vi "OP500ZP_SEALING.vi"(8 "ERRIN":errorcluster caption="entrée d'erreur (pas d'erreur)") -> (0 "ERROUT":errorcluster caption="sortie d'erreur", 2 "SEALING_VALUE":dbl, 3 "IsOK?":bool)   [LabVIEW 2020]
uses:
  VG/VG_ATEQ.vi
  <instrlib>/HIOKI BT356X Series/HIOKI BT356X Series.lvlib
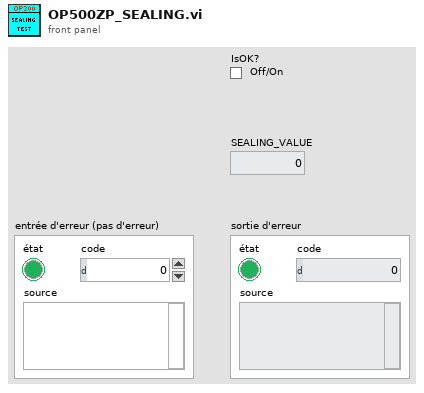
[diagram p1: front panel]
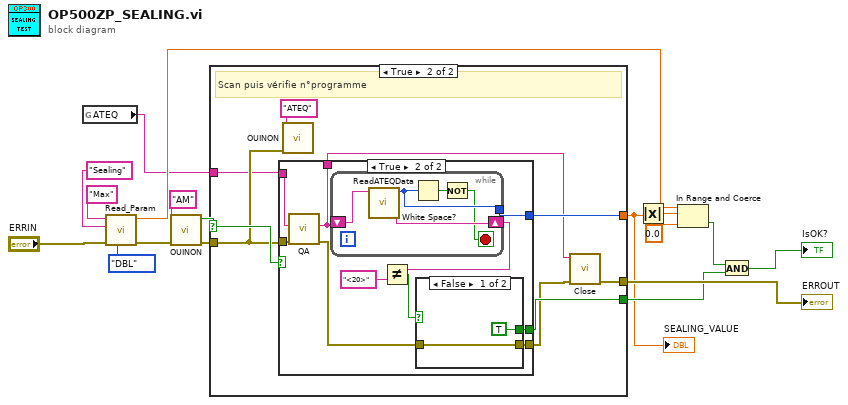
[diagram p0: block diagram]
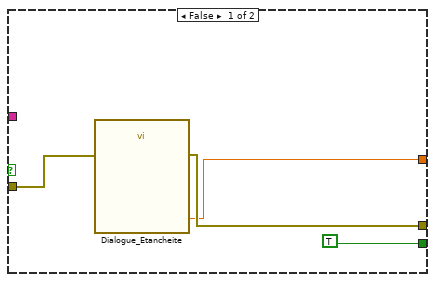
[diagram p2: hidden frame]
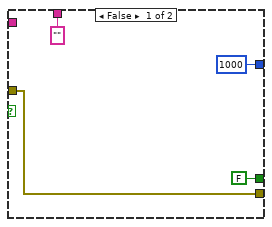
[diagram p3: hidden frame]
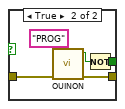
[diagram p4: hidden frame]
diagram:
  n1 = global read "VG_ATEQ.vi" "ATEQ"() -> (w1:string)
  n2 = call <userlib>:"Read_Param.vi"("Énum"=enum16{"STR", "DBL", "U32"}."DBL", "errin"="ERRIN", "section"="Sealing", "key"="Max") -> ("error out"=w7:errorcluster, "dbl"=w11:dbl)  [unwired: 3 in, 3 out]
  n3 = call <userlib>:"OUINON.vi"("errin"=w7, "image"="AM" ("IN")) -> ("error out"=w5:errorcluster, "OUI/NON"=w6:bool)  [unwired: 8 in]
  n4 = case shown="True" w6 {
    selector: w6 -> [_ w27]
    tunnel: [w20 w30] -> w3
    tunnel: [w21 w24] -> w16
    tunnel: [TRUE w29] -> w9
    tunnel: w5 -> [w18 w26]
    tunnel: w1 -> [_ w22]
    frame False {
      n5 = call "Dialogue_Etancheite.vi"("error in (no error)"=w18) -> ("Valeur d'étanchéité"=w20:dbl, "error out"=w21:errorcluster)  [unwired: 16 in, 1 out]
    }
    frame True {
      # "Scan puis vérifie n°programme"
      n6 = case shown="True" w27 {
        tunnel: [1000 ("Valeur") w44] -> w30
        tunnel: [w34 w42] -> w25
        tunnel: [FALSE w41] -> w29
        tunnel: w26 -> [w34 w37]
        tunnel: ["" ("DATAOUT") w36] -> w23
        tunnel: w22 -> [_ w35]
        frame False {
        }
        frame True {
          n7 = call "QA.vi"("ERRIN"=w37, "VISA"=w35) -> ("ERROUT"=w43:errorcluster, "DATAOUT"=w36:string)  [unwired: 8 in]
          n8 = while {
            tunnel: [w49] -> w44
            shift-right: [w47] -> w40
            shift-left: w36 -> [w48]
            stop <- w45 stop-if-true
            n9 = call "ReadATEQData.vi"("Chaîne"=w48) -> ("Prg number"=w47:string, "Valeur"=w49:i32)  [unwired: 7 in, 2 out]
            n10 = White Space?(1:w49) -> (0:w46:bool)
            n11 = Not(x=w46) -> (.not. x?=w45:bool)
          }
          n12 = Not Equal?(x=w40, y="<20>") -> (x != y?=w38:bool)
          n13 = case shown="False" w38 {
            tunnel: w43 -> [w50 w55]
            tunnel: [w50 w54] -> w42
            tunnel: [TRUE w52] -> w41
            frame False {
            }
            frame True {
              n14 = call <userlib>:"OUINON.vi"("errin"=w55, "image"="PROG" ("IN")) -> ("error out"=w54:errorcluster, "OUI/NON"=w53:bool)  [unwired: 8 in]
              n15 = Not(x=w53) -> (.not. x?=w52:bool)
            }
          }
        }
      }
      n16 = call <userlib>:"OUINON.vi"("errin"=w26, "image"="ATEQ" ("IN")) -> ()  [unwired: 8 in, 2 out]
      n17 = call <instrlib>:"Close.vi"("error in (no error)"=w25, "VISA resource name"=w23) -> ("error out"=w24:errorcluster)  [unwired: 9 in]
    }
  }
  "SEALING_VALUE" <- w3
  "ERROUT" <- w16
  n18 = Absolute Value(x=w3) -> (abs(x)=w2:dbl)
  n19 = In Range and Coerce ("Dans la gamme")(upper limit=w11, x=w2, lower limit=0.0 ("limite inférieure")) -> (In Range?=w10:bool)  [unwired: 1 out]
  n20 = And(x=w10, y=w9) -> (x .and. y?=→"IsOK?":bool)
